vi "Write Definitions.vi"(8 "error in (no error)":errorcluster, 10 "Definitions":T1={"External MemorySize"=32768, "Internal Memory Size"=512, "Overhead Ticks"=3, "Min Delay Loops"=3, "Loop Count Correction"=1, "Long Delay Loop Count Correction"=2, "Min Instruction Ticks"=6, "Long Delay Ticks"=4294967295, "Clock Period (s)"=1e-08, "Overhead Time (s)"=3e-08, "Min Instruction Cycle Time (s)"=9e-08, "Long Delay Time (s) "=42.94967298} {"Long Delay Time (s)" format="%.8p"; "Min Instruction Cycle Time (s)" format="%.0p"; "Overhead Time (s)" format="%.0p"; "Clock Period (s)" format="%.0p"; "Long Delay Ticks" format="%.0x"}, 11 "Slave_Pulseblaster in":refnum<class "Slave_Pulseblaster.lvclass">) -> (0 "error out":errorcluster, 3 "Slave_Pulseblaster out":refnum<class "Slave_Pulseblaster.lvclass">)   [LabVIEW 2013, in "Slave_Pulseblaster.lvclass"]
uses:
  Slave_Pulseblaster.lvclass
  Slave_Pulseblaster.lvclass/Slave_Pulseblaster.ctl
panel:
  # "(Period*Long D Ticks)+Overhead time"
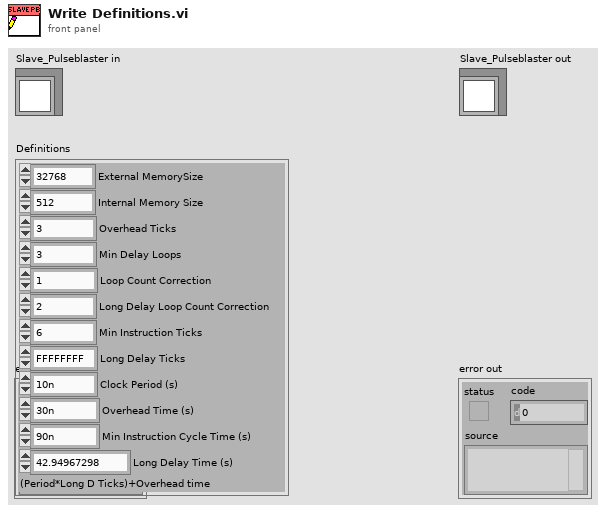
[diagram p1: front panel]
types:
  T1 = cluster{"External MemorySize":u16, "Internal Memory Size":u16, "Overhead Ticks":u8, "Min Delay Loops":u8, "Loop Count Correction":u8, "Long Delay Loop Count Correction":u8, "Min Instruction Ticks":u8, "Long Delay Ticks":u64, "Clock Period (s)":dbl, "Overhead Time (s)":dbl, "Min Instruction Cycle Time (s)":dbl, "Long Delay Time (s) ":dbl}
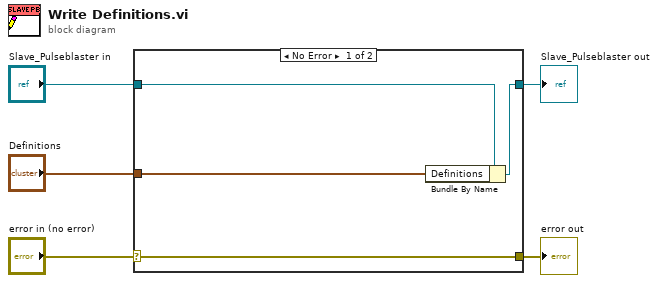
[diagram p0: block diagram]
diagram:
  n1 = case shown="No Error" "error in (no error)" {
    selector: "error in (no error)" -> [w9 w10]
    tunnel: [w9 w10] -> w4
    tunnel: [w7 w11] -> w2
    tunnel: "Slave_Pulseblaster in" -> [w8 w11]
    tunnel: "Definitions" -> [w6 _]
    frame No Error {
      n2 = Bundle By Name(cluster=w8, "Definitions"=w6) -> (w7:refnum<class "Slave_Pulseblaster.lvclass">)
    }
    frame Error {
    }
  }
  "error out" <- w4
  "Slave_Pulseblaster out" <- w2
